vi "Read MP Message.vi"(7 "Micropulse # In":i32, 8 "error in (no error)":errorcluster, 10 "data controls":T1={"Scan Reset"=FALSE, "Sub Sampling"=1, "Report Data Msg"=FALSE} {"Sub Sampling" items=["", "1:1", "2:1", "3:1", "4:1", "5:1", "6:1", "7:1", "8:1", "9:1", "10:1"]}) -> (0 "error out":errorcluster, 1 "message header":u16 format="%.0x", 2 "scan data info":T3 {"Error Message" format="%04x"; "Message Header" format="%04x"; "IP"."MIP location" format="%#.0f"; "IP"."Location" format="%#.0f"; "PRF" format="%.0fHz"}, 3 "Instrument Message":string, 5 "Micropulse # Out":i32)   [LabVIEW 2026, in "MicroPulse_Driver.lvlib"]
uses:
  MicroPulse_Driver.lvlib
  Datatypes/MP - scan data info.ctl
  Datatypes/MP - data output format.ctl
  Datatypes/MP - retain scan.ctl
  Datatypes/MP - axis positions (LLC).ctl
  Datatypes/MP - extracted data controls.ctl
  Datatypes/PNDT - subsampling.ctl
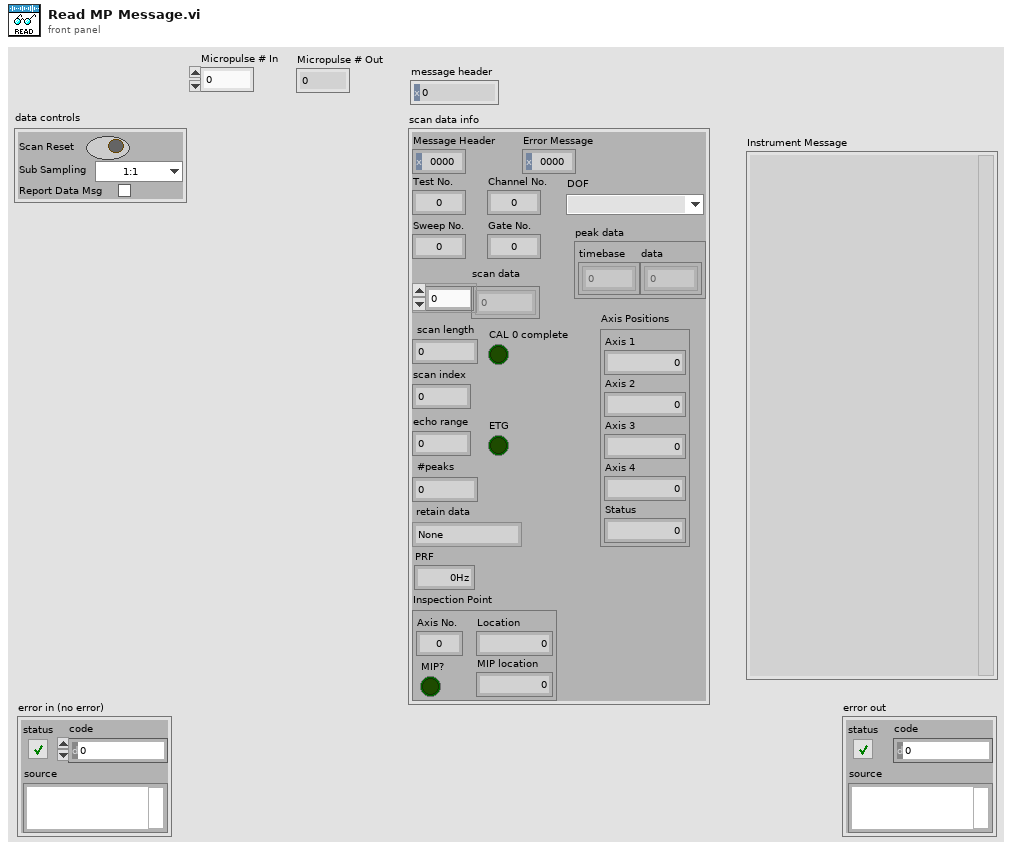
[diagram p1: front panel]
types:
  T1 = typedef "MicroPulse_Driver.lvlib/MP - extracted data controls.ctl" = cluster{"Scan Reset":bool, "Sub Sampling":T2, "Report Data Msg":bool}
  T2 = typedef "MicroPulse_Driver.lvlib/PNDT - subsampling.ctl" = u16
  T3 = typedef "MicroPulse_Driver.lvlib/MP - scan data info.ctl" = cluster{"Message Header":u16, "Error Message":u16, "Test No.":u32, "Channel No.":u8, "Sweep No.":u32, "Gate No.":u32, "DOF":T4, "retain data":T5, "scan data":u16[], "scan length":i32, "scan index":i32, "peak data":cluster{"timebase":u16[], "data":u16[]}, "#peaks":i32, "PRF":dbl, "IP":cluster{"Axis No.":u8, "Location":u32, "MIP location":u32, "MIP?":bool}, "echo range":u16, "ETG":bool, "CAL 0 complete":bool, "Axis Positions":T6}
  T4 = typedef "MicroPulse_Driver.lvlib/MP - data output format.ctl" = enum16{"", "8-bit Mode", "10-bit Mode", "12-bit Mode", "16-bit Mode", "8-bit Log Mode", "12-bit Packed Mode"}
  T5 = typedef "MicroPulse_Driver.lvlib/MP - retain scan.ctl" = enum16{"None", "Ascan", "Peaks"}
  T6 = typedef "MicroPulse_Driver.lvlib/MP - axis positions (LLC).ctl" = cluster{"Axis 1":u32, "Axis 2":u32, "Axis 3":u32, "Axis 4":u32, "Status":u8}
  T7 = typedef "MicroPulse_Driver.lvlib/MP-Registry Data-Cluster.ctl" = cluster{"Instrument Type":T8, "Serial #":u64, "Sample Frequency":T9, "dt (us)":dbl, "DOF":T4, "Material Velocity":dbl, "Asynch Reads":T10, "NUM of Tests":u32, "System Details":T11, "Gates":T13[], "Encoders":T20[], "CMD LUT":variant, "Command List":string}
  T8 = typedef "MicroPulse_Driver.lvlib/MP - instrument type.ctl" = enum16{"MicroPulse 5", "LT1", "LT2", "LTPA", "MPLT", "MicroPulse 6", "PipeScanner", "<MicroPulse>", "Micropulse 4", "Simulated Data"}
  T9 = typedef "MicroPulse_Driver.lvlib/MP - sample frequency.ctl" = enum16{"Use Default", "200MHz (LT2 only)", "100MHz", "50MHz", "25MHz", "10MHz"}
  T10 = typedef "MicroPulse_Driver.lvlib/MP - asynch read mode.ctl" = enum16{"Disabled", "Enabled"}
  T11 = typedef "MicroPulse_Driver.lvlib/MP - general system status.ctl" = cluster{"System Type":T8, "Serial No.":u64, "Channels":cluster{"Conv":u8, "PA":u16, "Extra":u32}, "Sample Frequency":cluster{"Default":u8, "Actual":u8}, "Software Versions":string, "Data Output Format":cluster{"Default":T4, "Actual":T4}, "Temperatures":cluster{"System":u8, "Processor":u8, "Slave Sys":u8, "Slave Proc":u8}, "Tx Buffer Size":u32, "System Error":string, "No. of Cards":u8, "DAC Gain":i16, "Uptimes":cluster{"since Power":u32, "since RSTS":u32, "since SRST":u32}, "Voltages":cluster{"Nominal":dbl, "Measured":dbl, "Difference":dbl}[], "Interface Cards":T12[]}
  T12 = typedef "MicroPulse_Driver.lvlib/MP - interface card status.ctl" = cluster{"Status":u8, "Map":u8, "Board - T":u8, "FPGA - T":u8, "PAIF Status":string, "Version":string}
  T13 = typedef "MicroPulse_Driver.lvlib/MP - Registry Gates.ctl" = cluster{"Display Gate":T14, "ETM Mode":T15, "Echo Gate":T16, "Insp Gates":T17[]}
  T14 = typedef "MicroPulse_Driver.lvlib/MP - display gate.ctl" = cluster{"Start":dbl, "Length":dbl}
  T15 = typedef "MicroPulse_Driver.lvlib/MP - echo gate mode.ctl" = enum16{"Echo Trigger OFF", "Echo Gate Display Mode", "Echo Trigger ON", "Multi Gate or FMC Mode", "Reserved", "PA - Echo Trigger ON"}
  T16 = typedef "MicroPulse_Driver.lvlib/MP - echo gate parameters.ctl" = cluster{"Start (us)":dbl, "Length (us)":dbl, "Threshold":u16, "Colour":u32}
  T17 = typedef "MicroPulse_Driver.lvlib/MP - multigate inspection gate parameters.ctl" = cluster{"Start (us)":dbl, "Length (us)":dbl, "Threshold":u16, "Enabled?":bool, "Max # Peaks":u16, "Hysteresis":T18, "Mode":T19, "Inverted?":bool, "Colour ":u32}
  T18 = typedef "MicroPulse_Driver.lvlib/MP - hysteresis level.ctl" = enum16{"None", "3dB", "6dB", "9dB", "12dB"}
  T19 = typedef "MicroPulse_Driver.lvlib/MP - multigate mode.ctl" = enum16{"1st Peak in Gate", "Largest Peak In Gate", "All Peaks In Gate", "1st Threshold Crossing"}
  T20 = typedef "MicroPulse_Driver.lvlib/MP - encoder settings.ctl" = cluster{"Encoder Type":T21, "Counts/mm":u32, "Enable Termination?":bool, "Multiplier":u32, "Backlash Period (s)":dbl, "Encoder Filter":u32}
  T21 = typedef "MicroPulse_Driver.lvlib/MP - encoder type.ctl" = enum16{"Quadrature", "Step/Direction"}
  T22 = typedef "MicroPulse_Driver.lvlib/TCP config.ctl" = cluster{"Connection ID":refnum<k5>, "IP address":string, "host port":u16, "OC timeout":i32, "Read timeout":i32, "Write timeout":i32}
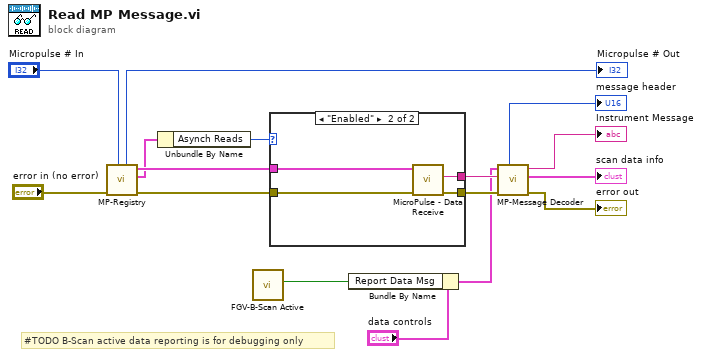
[diagram p0: block diagram]
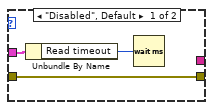
[diagram p2: hidden frame]
diagram:
  # "#TODO B-Scan active data reporting is for debugging only"
  n1 = call "MP-Registry.vi"("Micropulse # In"="Micropulse # In", "error in (no error)"="error in (no error)") -> ("error out"=w12:errorcluster, "Micropulse Data"=w7:T7, "TCP config"=w8:T22, "Micropulse # Out"=→"Micropulse # Out":i32)  [unwired: 6 in]
  n2 = Unbundle By Name(w7) -> ("Asynch Reads"=w4:T10)
  n3 = call "FGV-B-Scan Active.vi"() -> ("B-Scan Start?"=w2:bool)  [unwired: 9 in, 2 out]
  n4 = case shown="\"Enabled\"" w4 {
    tunnel: w12 -> [w19 w23]
    tunnel: w8 -> [w18 w22]
    tunnel: [w19 w21] -> w6
    tunnel: [_ w20] -> w5
    frame "Disabled", Default {
      n5 = Unbundle By Name(w18) -> ("Read timeout"=w17:i32)
      n6 = Wait (ms)(milliseconds to wait=w17) -> ()  [unwired: 1 out]
    }
    frame "Enabled" {
      n7 = call "MicroPulse - Data Receive.vi"("error in (no error)"=w23, "TCP config"=w22) -> ("error out"=w21:errorcluster, "data message"=w20:string)  [unwired: 4 in, 4 out]
    }
  }
  n8 = Bundle By Name(cluster="data controls", "Report Data Msg"=w2) -> (w1:T1)
  n9 = call "MP-Message Decoder.vi"("error in (no error)"=w6, "SDO messages"=w5, "data controls"=w1) -> ("error out"=→"error out":errorcluster, "scan data info"=→"scan data info":T3, "Instrument Message"=→"Instrument Message":string, "message header"=→"message header":u16)  [unwired: 2 in, 3 out]
